vi "Forward For inch.vi"(8 "Angle robot facing":dbl, 9 "Speed":dbl, 10 "Distance":dbl, 11 "RobotDriveDevRef in":T1) -> (3 "RobotDriveDevRef out":T1)   [LabVIEW 2015]
uses:
  <vilib>/Rock Robotics/WPI/RobotDrive/WPI_RobotDriveDevRef.ctl
  <vilib>/Rock Robotics/WPI/MotorControl/WPI_MotorControlDeviceRef.ctl
  <vilib>/Rock Robotics/WPI/MotorControl/WPI_MotorControlType.ctl
  <vilib>/Rock Robotics/SystemInterfaces/DIO/FPGA_DIOPWMChannel.ctl
  <vilib>/Rock Robotics/WPI/PWM/WPI_PWMDeadband.ctl
  <vilib>/Rock Robotics/WPI/CAN/Jaguar/SubVIs/WPI_CANJaguar_ControlMode.ctl
  <vilib>/Rock Robotics/WPI/CAN/TalonSRX/WPI_CANTalonSRX_APIControlMode.ctl
  <vilib>/Rock Robotics/WPI/RobotDrive/WPI_RobotDriveArcadeDrive_Standard(NoSaturation).vi
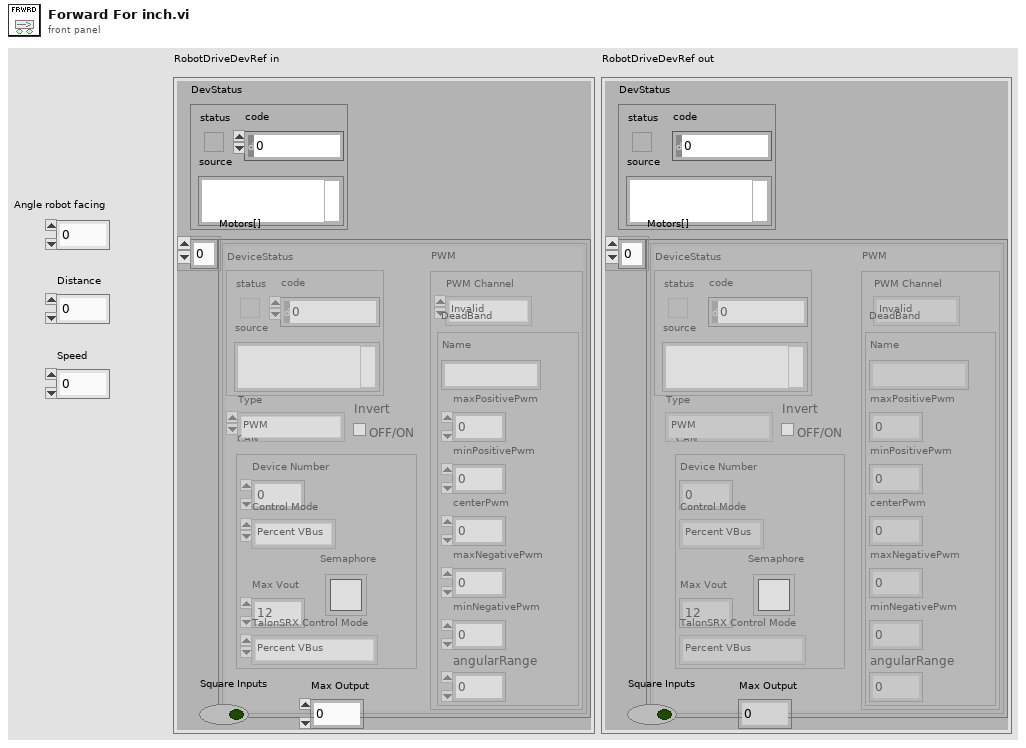
[diagram p1: front panel]
types:
  T1 = typedef "WPI_RobotDriveDevRef.ctl" = cluster{"DevStatus":errorcluster, "Motors[]":T2[], "Square Inputs":bool, "Max Output":dbl}
  T2 = typedef "WPI_MotorControlDeviceRef.ctl" = cluster{"DeviceStatus":errorcluster, "Type":T3, "PWM":cluster{"PWM Channel":T4, "DeadBand":T5}, "CAN":cluster{"Device Number":u8, "Control Mode":T6, "Semaphore":T7, "Max Vout":dbl, "TalonSRX Control Mode":T8}, "Invert":bool}
  T3 = typedef "WPI_MotorControlType.ctl" = enum16{"PWM", "CAN", "CANTalonSRX"}
  T4 = typedef "FPGA_DIOPWMChannel.ctl" = enum8{"PWM 0", "PWM 1", "PWM 2", "PWM 3", "PWM 4", "PWM 5", "PWM 6", "PWM 7", "PWM 8", "PWM 9", "PWM MXP 0", "PWM MXP 1", "PWM MXP 2", "PWM MXP 3", "PWM MXP 4", "PWM MXP 5", "PWM MXP 6", "PWM MXP 7", "PWM MXP 8", "PWM MXP 9", "Invalid"}
  T5 = typedef "WPI_PWMDeadband.ctl" = cluster{"Name":string, "maxPositivePwm":i32, "minPositivePwm":i32, "centerPwm":i32, "maxNegativePwm":i32, "minNegativePwm":i32, "angularRange":u16}
  T6 = typedef "WPI_CANJaguar_ControlMode.ctl" = enum8{"Percent VBus", "Current", "Speed", "Position", "Voltage"}
  T7 = typedef "Semaphore RefNum" = refnum<k1>
  T8 = typedef "WPI_CANTalonSRX_APIControlMode.ctl" = enum8{"Percent VBus", "Speed", "Position", "Slave", "Unchanged / Invalid", "Voltage Compensation", "Current", "Motion Profile"}
  T9 = typedef "WPI_PotentiometerDevRef.ctl" = cluster{"DevStatus":errorcluster, "Analog Channel":T10, "Invert Output":bool}
  T10 = typedef "FPGA_AIChannel.ctl" = enum8{"AI 0", "AI 1", "AI 2", "AI 3", "AI MXP 0", "AI MXP 1", "AI MXP 2", "AI MXP 3", "Invalid"}
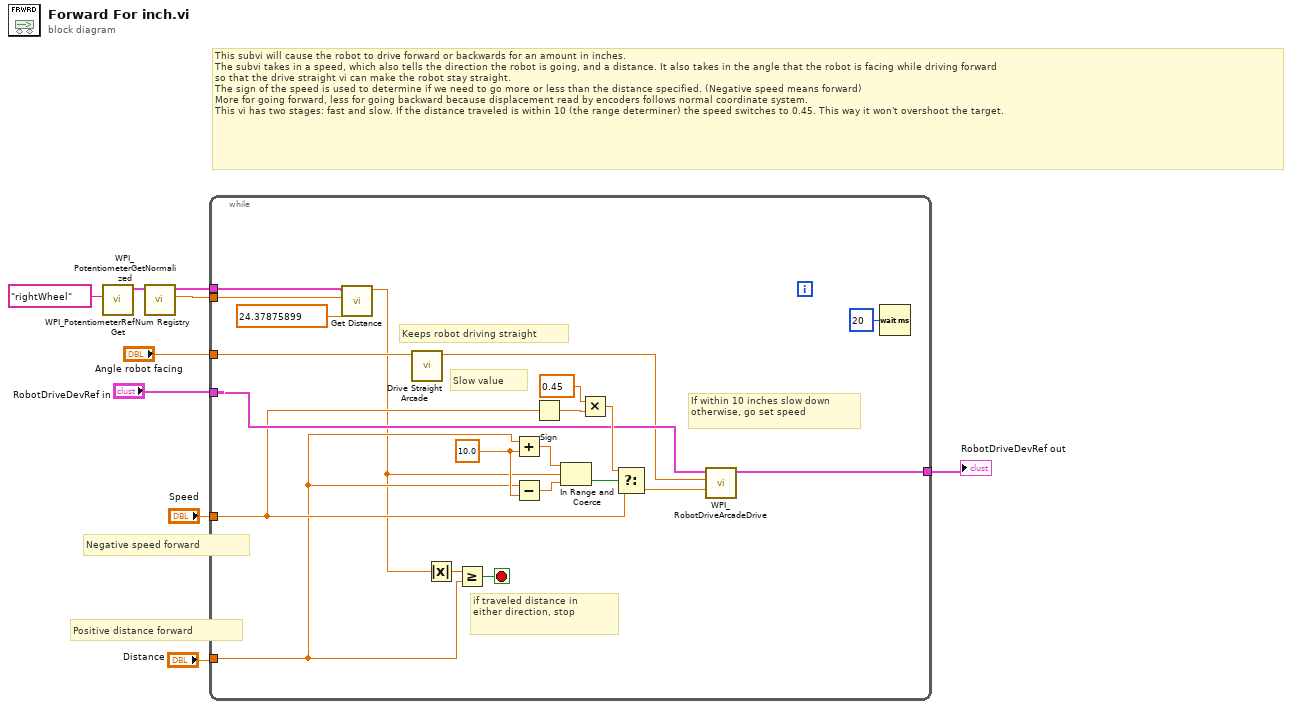
[diagram p0: block diagram]
diagram:
  # "Positive distance forward"
  # "Negative speed forward"
  # "This subvi will cause the robot to drive forward or backwards for an amount in inches.\nThe subvi takes in a speed, which also tells the direction the robot is going, and a distance. It also takes in the angle that the robot is facing while driving forward\nso that the drive straight vi can make the robot stay straight.\nThe sign of the speed is used to determine if we need to go more or less than the distance specified. (Negative speed means forward)\nMore for going forward, less for going backward because displacement read by encoders follows normal coordinate system. \nThis vi has two stages: fast and slow. If the distance traveled is within 10 (the range determiner) the speed switches to 0.45. This way it won't overshoot the target."
  n1 = call <vilib>:"WPI_PotentiometerRefNum Registry Get.vi"("refnum name"="rightWheel") -> ("PotDevRef"=w4:T9)  [unwired: 9 in, 1 out]
  n2 = call <vilib>:"WPI_PotentiometerGetNormalized.vi"("PotDevRef"=w4) -> ("Normalized Value"=w3:dbl, "PotDevRef"=w1:T9)  [unwired: 8 in, 1 out]
  n3 = while {
    tunnel: "RobotDriveDevRef in" -> [w22]
    tunnel: [w21] -> w2
    tunnel: "Distance" -> [w12]
    tunnel: "Speed" -> [w17]
    tunnel: "Angle robot facing" -> [w20]
    tunnel: w3 -> [w16]
    tunnel: w1 -> [w14]
    stop <- w11 stop-if-true
    w28 = 10.0
    # "if traveled distance in\neither direction, stop"
    # "If within 10 inches slow down\notherwise, go set speed"
    # "Keeps robot driving straight"
    # "Slow value"
    n4 = call "Get Distance.vi"("distance/rotation"=24.37875899 ("x"), "Starting value"=w16, "PotDevRef"=w14) -> ("Distance"=w10:dbl)  [unwired: 8 in]
    n5 = call "Drive Straight Arcade.vi"("Angle robot facing"=w20) -> ("Arcade drive x"=w19:dbl)  [unwired: 10 in]
    n6 = Absolute Value(x=w10) -> (abs(x)=w13:dbl)
    n7 = Greater Or Equal?(x=w13, y=w12) -> (x >= y?=w11:bool)
    n8 = Add(x=w12, y=w28) -> (x+y=w26:dbl)
    n9 = Subtract(x=w12, y=w28) -> (x-y=w27:dbl)
    n10 = Sign(1:w17) -> (0:w24:dbl)
    n11 = In Range and Coerce(upper limit=w26, x=w10, lower limit=w27) -> (In Range?=w29:bool)  [unwired: 1 out]
    n12 = Multiply(x=0.45 ("t"), y=w24) -> (x*y=w23:dbl)
    n13 = Select(t=w23, s=w29, f=w17) -> (s? t:f=w18:dbl)
    n14 = call-poly <vilib>:"WPI_RobotDriveArcadeDrive.vi"("Y axis value"=w18, "X axis value"=w19, "RobotDriveDevRef"=w22) -> ("RobotDriveDevRef"=w21:T1)  [unwired: 6 in, 2 out]
    n15 = Wait (ms)(milliseconds to wait=u32 20) -> ()  [unwired: 1 out]
  }
  "RobotDriveDevRef out" <- w2
